vi "saveDataNodeBegin.vi"(8 "error in (no error)":errorcluster, 9 "indent":i32, 10 "XML Refnum in":refnum<file>, 11 "Parameter in":refnum<class "Parameter.lvclass">) -> (0 "error out":errorcluster, 2 "XML Refnum out":refnum<file>, 3 "Parameter out":refnum<class "Parameter.lvclass">)   [LabVIEW 2013, in "Parameter.lvclass"]
doc: "Begins the process of saving a xceData Node to an XML formatted file."
uses:
  Parameter.lvclass
  channel_dataType.ctl
  Parameter.lvclass/Parameter.ctl
  xCE/xceDataNode/xceDataNode.lvclass
panel:
  in  "Data Type":T1
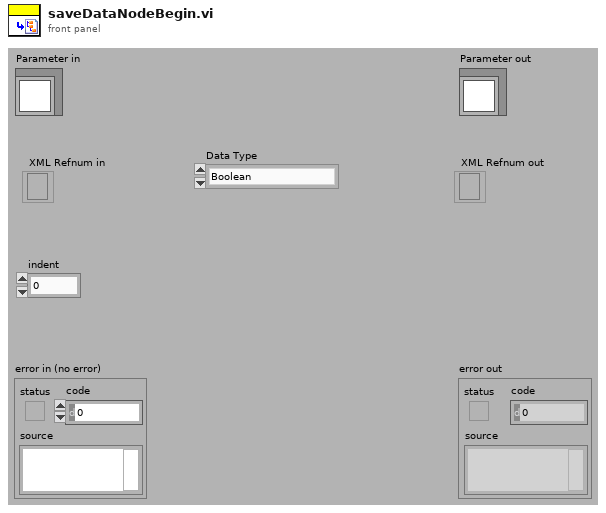
[diagram p1: front panel]
types:
  T1 = typedef "Parameter.lvclass/channel_dataType.ctl" = enum16{"Boolean", "U8", "I8", "U16", "I16", "U32", "I32", "U64", "I64", "FXPI32", "FXPU32", "FXPI64", "FXPU64", "PWM"}
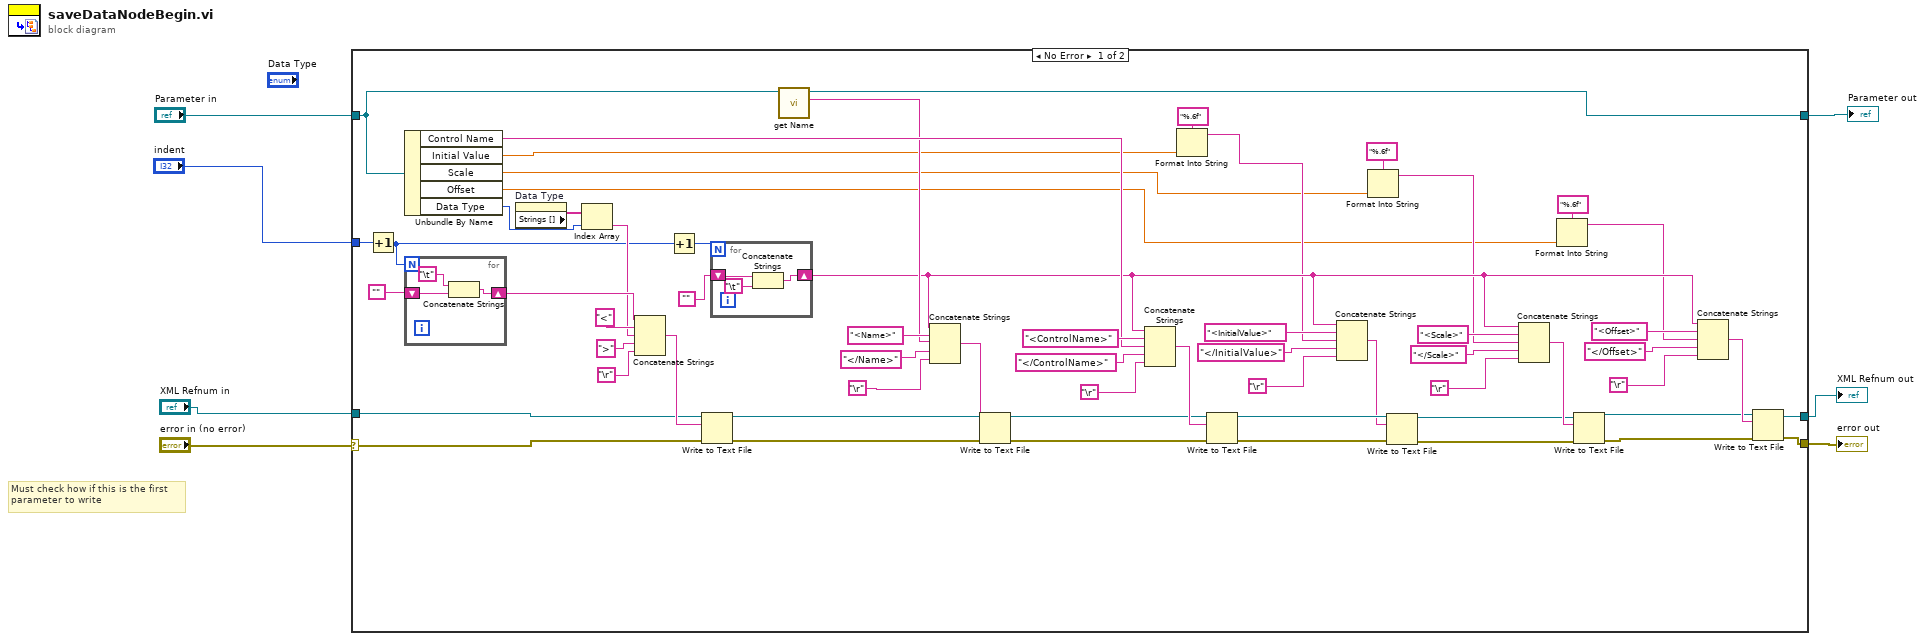
[diagram p0: block diagram]
diagram:
  # "Must check how if this is the first\nparameter to write"
  n1 = case shown="No Error" "error in (no error)" {
    selector: "error in (no error)" -> [w44 w76]
    tunnel: "Parameter in" -> [w35 w77]
    tunnel: [w34 w77] -> w7
    tunnel: [w20 w76] -> w5
    tunnel: [w21 w75] -> w6
    tunnel: "XML Refnum in" -> [w42 w75]
    tunnel: "indent" -> [w37 _]
    frame No Error {
      n2 = Increment(x=w37) -> (x+1=w38:i32)
      n3 = Unbundle By Name(w35) -> ("Control Name"=w50:string, "Initial Value"=w16:dbl, "Scale"=w11:dbl, "Offset"=w9:dbl, "Data Type"=w40:T1)
      n4 = for {
        N: w38 -> [_]
        shift-right: [w71] -> w45
        shift-left: "" -> [w70]
        n5 = Concatenate Strings("\t", w70) -> (w71:string)
      }
      n6 = property on="Data Type" class="Enum (strict)"() -> ("Strings []"=w41:string[])  [unwired: 2 in, 2 out]
      n7 = Index Array(array=w41, index=w40) -> (element=w39:string)
      n8 = Concatenate Strings(w45, "<", w39, ">", "\r") -> (w43:string)
      n9 = Increment(x=w38) -> (x+1=w67:i32)
      n10 = Write to Text File(file (use dialog)=w42, text=w43, error in=w44) -> (refnum out=w29:refnum<file>, error out=w27:errorcluster)  [unwired: 1 in, 1 out]
      n11 = for {
        N: w67 -> [_]
        shift-right: [w72] -> w17
        shift-left: "" -> [w74]
        n12 = Concatenate Strings(w74, "\t") -> (w72:string)
      }
      n13 = call "get Name.vi"("xceDataNode in"=w35) -> ("Name"=w33:string, "xceDataNode out"=w34:refnum<class "Parameter.lvclass">)  [unwired: 8 in, 1 out]
      n14 = Concatenate Strings(w17, "<Name>" ("string"), w33, "</Name>" ("string"), "\r") -> (w30:string)
      n15 = Write to Text File(file (use dialog)=w29, text=w30, error in=w27) -> (refnum out=w28:refnum<file>, error out=w26:errorcluster)  [unwired: 1 in, 1 out]
      n16 = Concatenate Strings(w17, "<ControlName>" ("string"), w50, "</ControlName>" ("string"), "\r") -> (w62:string)
      n17 = Format Into String(format string="%.6f", w16) -> (resulting string=w15:string)  [unwired: 2 in, 1 out]
      n18 = Write to Text File(file (use dialog)=w28, text=w62, error in=w26) -> (refnum out=w58:refnum<file>, error out=w53:errorcluster)  [unwired: 1 in, 1 out]
      n19 = Concatenate Strings(w17, "<InitialValue>" ("string"), w15, "</InitialValue>" ("string"), "\r") -> (w54:string)
      n20 = Format Into String(format string="%.6f", w11) -> (resulting string=w10:string)  [unwired: 2 in, 1 out]
      n21 = Write to Text File(file (use dialog)=w58, text=w54, error in=w53) -> (refnum out=w59:refnum<file>, error out=w52:errorcluster)  [unwired: 1 in, 1 out]
      n22 = Concatenate Strings(w17, "<Scale>" ("string"), w10, "</Scale>" ("string"), "\r") -> (w63:string)
      n23 = Format Into String(format string="%.6f", w9) -> (resulting string=w8:string)  [unwired: 2 in, 1 out]
      n24 = Write to Text File(file (use dialog)=w59, text=w63, error in=w52) -> (refnum out=w18:refnum<file>, error out=w19:errorcluster)  [unwired: 1 in, 1 out]
      n25 = Concatenate Strings(w17, "<Offset>" ("string"), w8, "</Offset>" ("string"), "\r") -> (w25:string)
      n26 = Write to Text File(file (use dialog)=w18, text=w25, error in=w19) -> (refnum out=w21:refnum<file>, error out=w20:errorcluster)  [unwired: 1 in, 1 out]
    }
    frame Error {
    }
  }
  "error out" <- w5
  "Parameter out" <- w7
  "XML Refnum out" <- w6
